vi "Glyph Transform.vi"(8 "error in (no error)":errorcluster, 9 "Offset":cluster{"x":sgl, "y":sgl}, 10 "Matrix":T1=[[1.0, 0.0], [0.0, 1.0]], 11 "glyph ref":i64) -> (0 "error out":errorcluster, 3 "glyph ref":i64)   [LabVIEW 2023, in "Freetype Drawer.lvlib"]
uses:
  Freetype Drawer.lvlib
  <vilib>/Analysis/Matrix/Datatypes/RealMatrix.ctl
  libfreetype.dll
  <vilib>/Analysis/Matrix/NI_Matrix.lvlib
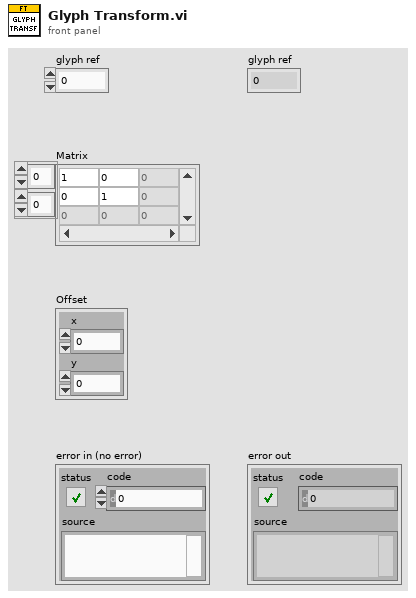
[diagram p1: front panel]
types:
  T1 = typedef "NI_Matrix.lvlib/RealMatrix.ctl" = dbl[][]
  T2 = cluster{"Matrix[0]":dbl, "Matrix[1]":dbl, "Matrix[2]":dbl, "Matrix[3]":dbl}
  T3 = cluster{"Matrix[0]":i32, "Matrix[1]":i32, "Matrix[2]":i32, "Matrix[3]":i32}
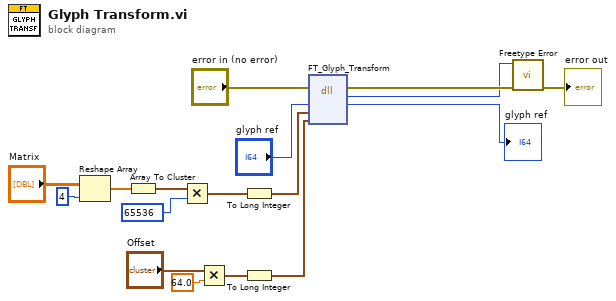
[diagram p0: block diagram]
diagram:
  n1 = Reshape Array("Matrix", 4 ("dimension size")) -> (w7:dbl[])
  n2 = Array To Cluster(array=w7) -> (cluster=w5:T2)
  n3 = Multiply(x=w5, y=65536) -> (x*y=w11:T2)
  n4 = Multiply(x="Offset", y=sgl 64.0) -> (x*y=w12:cluster{"x":sgl, "y":sgl})
  n5 = To Long Integer(number=w11) -> (32bit integer=w9:T3)
  n6 = To Long Integer(number=w12) -> (32bit integer=w1:cluster{"x":i32, "y":i32})
  n7 = dll-call lib="E:/Labview/LV 2023/Libs/LV Symbol/Freetype Drawer/libfreetype.dll" fn="FT_Glyph_Transform"(error in="error in (no error)", "face"="glyph ref", "matrix"=w9, "delta"=w1) -> (error out=w14:errorcluster, "error"=w2:i32, "face"=→"glyph ref":i64)  [unwired: 4 in, 1 out]
  n8 = call "Freetype Error.vi"("error in (no error)"=w14, "Error"=w2) -> ("error out"=→"error out":errorcluster)  [unwired: 9 in]
